vi "Self Event Alias.vi"(11 "Hello World Event in":refnum<class "Hello World Event.lvclass">) -> (2 "Self Event Alias":string)   [LabVIEW 2021, in "Hello World Event.lvlib" / "Hello World Event.lvclass"]
uses:
  Hello World Event.lvclass
  Hello World Event.lvclass/Hello World Event.ctl
  jettl/Event jettl/Event jettl.lvclass
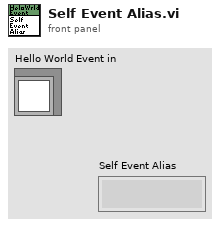
[diagram p1: front panel]
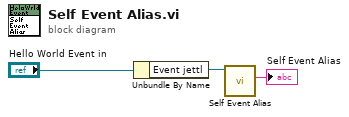
[diagram p0: block diagram]
diagram:
  n1 = Unbundle By Name("Hello World Event in") -> ("Event jettl"=w2:refnum<class "Event jettl.lvclass">)
  n2 = call-dynamic "Self Event Alias.vi"("Event jettl in"=w2) -> ("Self Event Alias"=→"Self Event Alias":string)  [unwired: 10 in]
